vi "Lab Panel V4.85.vi"() -> ()   [LabVIEW 2013] (continued)
                  frame True {
                    n2927 = Multiply(x=w5340, y=w5339) -> (x*y=w5338:dbl)
                    n2928 = Multiply(x=w5340, y=w5342) -> (x*y=w5341:dbl)
                  }
                }
                n2929 = local read "SIG LAB05-1"() -> (w5327:T2)
                n2930 = Bundle By Name(cluster=w5327, "Tmp Live"=w5307, "Tmp Neut"=w5306) -> (w5326:T2)
                n2931 = local read "SIG LAB05-2"() -> (w5325:T2)
                n2932 = Bundle By Name(cluster=w5325, "Tmp Live"=w5303, "Tmp Neut"=w5302) -> (w5324:T2)
                n2933 = local write "SIG LAB05-1"(w5326) -> ()
                n2934 = local write "SIG LAB05-2"(w5324) -> ()
              }
            }
          }
          frame #20 {
            # "write data to display panel"
            n2935 = global write "Global display 1.vi" "TEST 5-2"(w5359) -> ()
            n2936 = global write "Global display 1.vi" "TEST 4-2"(w5361) -> ()
            n2937 = global write "Global display 1.vi" "TEST 1-2"(w5367) -> ()
            n2938 = global write "Global display 1.vi" "TEST 3-1"(w5364) -> ()
            n2939 = global write "Global display 1.vi" "TEST 5-1"(w5360) -> ()
            n2940 = global write "Global display 1.vi" "TEST 1-1"(w5368) -> ()
            n2941 = global write "Global display 1.vi" "TEST 3-2"(w5363) -> ()
            n2942 = global write "Global display 1.vi" "TEST 4-1"(w5362) -> ()
            n2943 = global write "Global display 1.vi" "TEST 2-2"(w5365) -> ()
            n2944 = global write "Global display 1.vi" "TEST 2-1"(w5366) -> ()
            n2945 = global read "Global display 3.vi" "log 1-1"() -> (→"LOG LAB01-1":string)
            n2946 = global read "Global display 3.vi" "log 3-1"() -> (→"LOG LAB03-1":string)
            n2947 = global read "Global display 3.vi" "log 1-2"() -> (→"LOG LAB01-2":string)
            n2948 = property on="Tab Control 2" class="TabCtl (strict)"() -> ("Pages"=w5358:refnum<vi>[])  [unwired: 2 in, 2 out]
            n2949 = global read "Global display 3.vi" "log 2-1"() -> (→"LOG LAB02-1":string)
            n2950 = global read "Global display 3.vi" "log 2-2"() -> (→"LOG LAB02-2":string)
            n2951 = global read "Global display 3.vi" "log 4-2"() -> (→"LOG LAB04-2":string)
            n2952 = global read "Global display 3.vi" "log 5-2"() -> (→"LOG LAB05-2":string)
            n2953 = global read "Global display 3.vi" "log 5-1"() -> (→"LOG LAB05-1":string)
            n2954 = global read "Global display 3.vi" "log 4-1"() -> (→"LOG LAB04-1":string)
            n2955 = global read "Global display 3.vi" "log 3-2"() -> (→"LOG LAB03-2":string)
            n2956 = Index Array(array=w5358, index=9) -> (element=w5356:refnum<vi>)
            n2957 = property class="Page"(reference=w5356) -> ("PageVis"=w5355:bool)  [unwired: 1 in, 2 out]
            n2958 = global write "Global display 3.vi" "admin"(w5355) -> ()
            n2959 = local read "O/I  LAB05-2"() -> (w5409:bool)
            n2960 = local read "O/I  LAB05-1"() -> (w5410:bool)
            n2961 = local read "O/I  LAB03-2"() -> (w5413:bool)
            n2962 = local read "O/I  LAB04-2"() -> (w5411:bool)
            n2963 = local read "O/I  LAB04-1"() -> (w5412:bool)
            n2964 = local read "O/I  LAB03-1"() -> (w5414:bool)
            n2965 = local read "O/I  LAB01-2"() -> (w5417:bool)
            n2966 = local read "O/I  LAB01-1"() -> (w5418:bool)
            n2967 = local read "O/I  LAB02-1"() -> (w5416:bool)
            n2968 = local read "O/I  LAB02-2"() -> (w5415:bool)
            n2969 = global write "Global display 1.vi" "5-2 O/F"(w5409) -> ()
            n2970 = global write "Global display 1.vi" "5-1 O/F"(w5410) -> ()
            n2971 = global write "Global display 1.vi" "4-1 O/F"(w5412) -> ()
            n2972 = global write "Global display 1.vi" "4-2 O/F"(w5411) -> ()
            n2973 = global write "Global display 1.vi" "3-2 O/F"(w5413) -> ()
            n2974 = global write "Global display 1.vi" "3-1 O/F"(w5414) -> ()
            n2975 = global write "Global display 1.vi" "2-2 O/F"(w5415) -> ()
            n2976 = global write "Global display 1.vi" "2-1 O/F"(w5416) -> ()
            n2977 = global write "Global display 1.vi" "1-2 O/F"(w5417) -> ()
            n2978 = global write "Global display 1.vi" "1-1 O/F"(w5418) -> ()
            n2979 = local read "run lab05-2"() -> (w5399:bool)
            n2980 = local read "run lab04-1"() -> (w5402:bool)
            n2981 = local read "run lab04-2"() -> (w5401:bool)
            n2982 = local read "run lab05-1"() -> (w5400:bool)
            n2983 = local read "run lab03-2"() -> (w5403:bool)
            n2984 = local read "run lab02-1"() -> (w5406:bool)
            n2985 = local read "run lab03-1"() -> (w5404:bool)
            n2986 = local read "run lab01-2"() -> (w5407:bool)
            n2987 = local read "run lab02-2"() -> (w5405:bool)
            n2988 = local read "run lab01-1"() -> (w5408:bool)
            n2989 = global write "Global display 1.vi" "5-2 R/S"(w5399) -> ()
            n2990 = global write "Global display 1.vi" "5-1 R/S"(w5400) -> ()
            n2991 = global write "Global display 1.vi" "4-2 R/S"(w5401) -> ()
            n2992 = global write "Global display 1.vi" "4-1 R/S"(w5402) -> ()
            n2993 = global write "Global display 1.vi" "3-2 R/S"(w5403) -> ()
            n2994 = global write "Global display 1.vi" "1-2 R/S"(w5407) -> ()
            n2995 = global write "Global display 1.vi" "2-1 R/S"(w5406) -> ()
            n2996 = global write "Global display 1.vi" "3-1 R/S"(w5404) -> ()
            n2997 = global write "Global display 1.vi" "2-2 R/S"(w5405) -> ()
            n2998 = global write "Global display 1.vi" "1-1 R/S"(w5408) -> ()
            n2999 = local read "DISP LAB04-2"() -> (w5391:T4)
            n3000 = local read "DISP LAB05-1"() -> (w5390:T4)
            n3001 = local read "DISP LAB04-1"() -> (w5392:T4)
            n3002 = local read "DISP LAB05-2"() -> (w5389:T4)
            n3003 = local read "DISP LAB03-1"() -> (w5394:T4)
            n3004 = local read "DISP LAB03-2"() -> (w5393:T4)
            n3005 = local read "DISP LAB01-2"() -> (w5397:T4)
            n3006 = local read "DISP LAB02-1"() -> (w5396:T4)
            n3007 = local read "DISP LAB02-2"() -> (w5395:T4)
            n3008 = local read "DISP LAB01-1"() -> (w5398:T4)
            n3009 = global write "Global display 2.vi" "DISP LAB05-1"(w5390) -> ()
            n3010 = global write "Global display 2.vi" "DISP LAB05-2"(w5389) -> ()
            n3011 = global write "Global display 2.vi" "DISP LAB04-2"(w5391) -> ()
            n3012 = global write "Global display 2.vi" "DISP LAB02-1"(w5396) -> ()
            n3013 = global write "Global display 2.vi" "DISP LAB02-2"(w5395) -> ()
            n3014 = global write "Global display 2.vi" "DISP LAB04-1"(w5392) -> ()
            n3015 = global write "Global display 2.vi" "DISP LAB01-2"(w5397) -> ()
            n3016 = global write "Global display 2.vi" "DISP LAB01-1"(w5398) -> ()
            n3017 = global write "Global display 2.vi" "DISP LAB03-1"(w5394) -> ()
            n3018 = global write "Global display 2.vi" "DISP LAB03-2"(w5393) -> ()
            n3019 = local read "SET LAB05-2"() -> (w5379:T5)
            n3020 = local read "SET LAB05-1"() -> (w5380:T5)
            n3021 = local read "SET LAB04-1"() -> (w5382:T5)
            n3022 = local read "SET LAB04-2"() -> (w5381:T5)
            n3023 = local read "SET LAB03-1"() -> (w5384:T5)
            n3024 = local read "SET LAB03-2"() -> (w5383:T5)
            n3025 = local read "SET LAB02-2"() -> (w5385:T5)
            n3026 = local read "SET LAB01-2"() -> (w5387:T5)
            n3027 = local read "SET LAB02-1"() -> (w5386:T5)
            n3028 = local read "SET LAB01-1"() -> (w5388:T5)
            n3029 = global write "Global display 2.vi" "SET LAB05-2"(w5379) -> ()
            n3030 = global write "Global display 2.vi" "SET LAB05-1"(w5380) -> ()
            n3031 = global write "Global display 2.vi" "SET LAB04-1"(w5382) -> ()
            n3032 = global write "Global display 2.vi" "SET LAB04-2"(w5381) -> ()
            n3033 = global write "Global display 2.vi" "SET LAB03-2"(w5383) -> ()
            n3034 = global write "Global display 2.vi" "SET LAB02-2"(w5385) -> ()
            n3035 = global write "Global display 2.vi" "SET LAB03-1"(w5384) -> ()
            n3036 = global write "Global display 2.vi" "SET LAB01-2"(w5387) -> ()
            n3037 = global write "Global display 2.vi" "SET LAB01-1"(w5388) -> ()
            n3038 = global write "Global display 2.vi" "SET LAB02-1"(w5386) -> ()
            n3039 = local read "RESULT LAB01-1"() -> (w5378:bool)
            n3040 = local read "RESULT LAB03-2"() -> (w5373:bool)
            n3041 = local read "RESULT LAB04-1"() -> (w5372:bool)
            n3042 = local read "RESULT LAB04-2"() -> (w5371:bool)
            n3043 = local read "RESULT LAB02-2"() -> (w5375:bool)
            n3044 = local read "RESULT LAB01-2"() -> (w5377:bool)
            n3045 = local read "RESULT LAB02-1"() -> (w5376:bool)
            n3046 = local read "RESULT LAB03-1"() -> (w5374:bool)
            n3047 = local read "RESULT LAB05-1"() -> (w5370:bool)
            n3048 = local read "RESULT LAB05-2"() -> (w5369:bool)
            n3049 = global write "Global display 2.vi" "RESULT LAB05-1"(w5370) -> ()
            n3050 = global write "Global display 2.vi" "RESULT LAB01-2"(w5377) -> ()
            n3051 = global write "Global display 2.vi" "RESULT LAB03-2"(w5373) -> ()
            n3052 = global write "Global display 2.vi" "RESULT LAB04-1"(w5372) -> ()
            n3053 = global write "Global display 2.vi" "RESULT LAB04-2"(w5371) -> ()
            n3054 = global write "Global display 2.vi" "RESULT LAB05-2"(w5369) -> ()
            n3055 = global write "Global display 2.vi" "RESULT LAB03-1"(w5374) -> ()
            n3056 = global write "Global display 2.vi" "RESULT LAB02-1"(w5376) -> ()
            n3057 = global write "Global display 2.vi" "RESULT LAB02-2"(w5375) -> ()
            n3058 = global write "Global display 2.vi" "RESULT LAB01-1"(w5378) -> ()
          }
          frame #21 {
            # "end main and display program"
            n3059 = Quit LabVIEW(quit? (T)="stop all") -> ()
            n3060 = global write "Global display 1.vi" "stop disp"("stop all") -> ()
          }
        }
        n3061 = node-c288() -> ()  [unwired: 1 in, 1 out]
        "loops" <- w291
      }
      n3062 = node-c288(w268) -> ()  [unwired: 1 out]
    }
  }
